vi "Init with SQL Record.vi"(8 "error in (no error)":errorcluster, 10 "MySQL Record":variant[](array[variant]), 11 "Credit Transaction in":refnum<class "Credit Transaction.lvclass">) -> (0 "error out":errorcluster, 3 "Credit Transaction out":refnum<class "Credit Transaction.lvclass">)   [LabVIEW 2018, in "Credit Transaction.lvclass"]
uses:
  Credit Transaction.lvclass
  Transaction/Transaction.lvclass
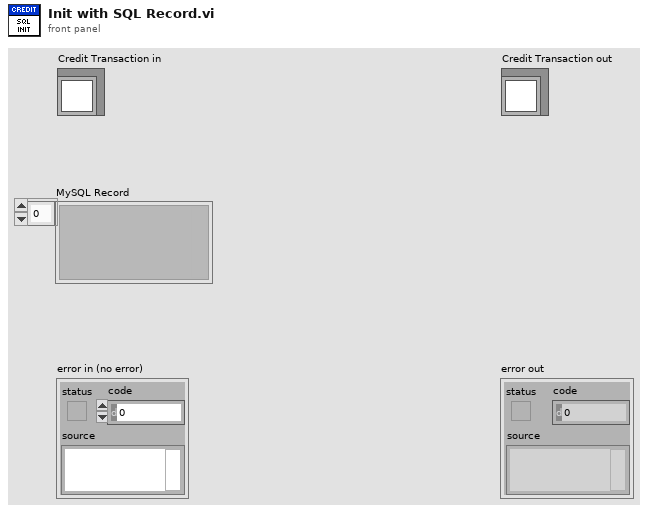
[diagram p1: front panel]
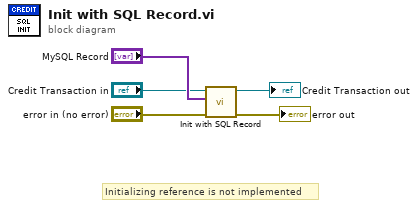
[diagram p0: block diagram]
diagram:
  # "Initializing reference is not implemented"
  n1 = call-parent "Init with SQL Record.vi"("error in (no error)"="error in (no error)", "MySQL Record"="MySQL Record", "Transaction in"="Credit Transaction in") -> ("error out"=→"error out":errorcluster, "Transaction out"=→"Credit Transaction out":refnum<class "Credit Transaction.lvclass">)  [unwired: 7 in]
